vi "타입캐스터.vi"() -> ()   [LabVIEW 2014]
panel:
  out "숫자 2":dbl format="%#_15g"
  out "길이 2":i32
  out "*(타입 *) &x":string
  out "숫자":dbl format="%#_15g"
  out "길이":i32
  out "F포맷 문자열":string
  out "숫자형":dbl format="%#_15f"
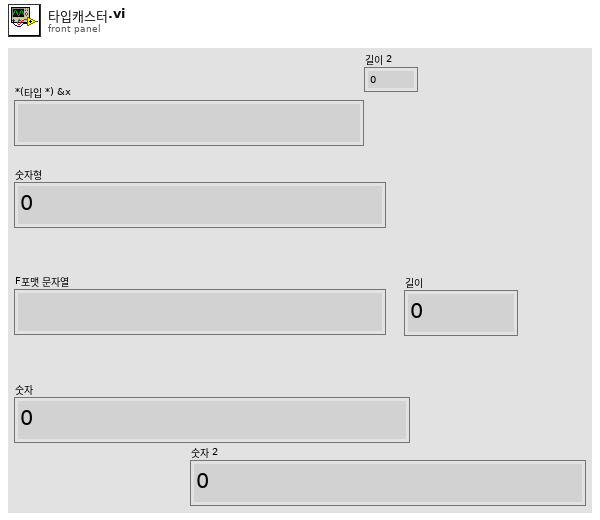
[diagram p1: front panel]
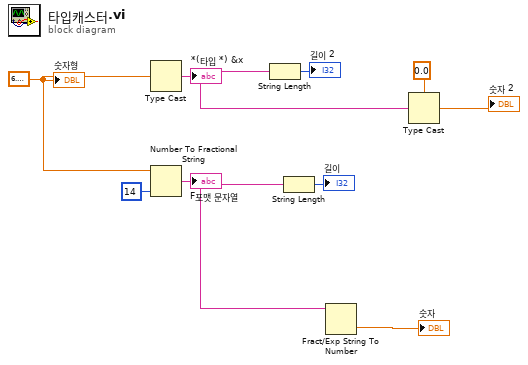
[diagram p0: block diagram]
diagram:
  w5 = 6.283185307179586
  n1 = Type Cast(x=w5) -> (*(type *) &x=w3:string)  [unwired: 1 in]
  "*(타입 *) &x" <- w3
  n2 = Number To Fractional String(number=w5, precision (6)=i16 14 ("정밀도(6)")) -> (F-format string=w7:string)  [unwired: 2 in]
  "F포맷 문자열" <- w7
  n3 = String Length(string=w3) -> (length=→"길이 2":i32)
  n4 = String Length(string=w7) -> (length=→"길이":i32)
  n5 = Fract/Exp String To Number(string=w7) -> (number=→"숫자":dbl)  [unwired: 3 in, 1 out]
  n6 = Type Cast(type=0.0, x=w3) -> (*(type *) &x=→"숫자 2":dbl)
  "숫자형" <- w5
